vi "Public Key File Authentication.vi"() -> ()   [LabVIEW 2018]
doc: "Logs into a remote SSH server using a username, Public-Private Key pair, and passphrase if the Public Key was created with one. This is arguably a more secure form of authentication than Password Authenication, but it requires configuration on the remote SSH server and/or CompactRIO."
uses:
  Toolkit/Session/Type Definitions/Host Key Hash Types.ctl
  Toolkit/Session/Support/Create from SSH.vi
  Toolkit/Session/Support/Destroy to SSH.vi
  Toolkit/SSH/SSH.lvclass
  Toolkit/Session/Session.lvclass
panel:
  in  "Private Key File":path
  in  "Public Key File":path
  out "Remote Host Key Type":string
  out "Remote Host Key":string
  out "Remote Fingerprint Hash":string
  out "Authenticated":bool
  in  "Remote SSH Server":string
  in  "Passphrase":string
  in  "Username":string
  # "Overview: Demonstrates transferring, or uploading, a local file to a remote SSH server, similar to the SCP command line utility\nInstructions:\n1. Enter the IP address or host name of the remote SSH server. This can be a CompactRIO (cRIO) running the National Instruments Linux Real-Time (NI Linux RT) operating system with the Enable Secure Shell Server (sshd) checkbox checked. \n2. Select a Public Key on the local computer.\n3. Select the Private Key sibling to the Public Key. Note, the Private Key should be private and only accessible by the current, local user. It is best practice to have permissions for the Private Key file be only read/write accessible by the local user and no one else. It is even better to use a key store application for storage of Public-Private Key pairs.\n4. Enter a username. If using a cRIO with a default configuration, then the username is \"admin\".\n5. Enter a passphrase if the Public Key was created with one. Note, it is best practice to always create a public key with a passphrase, then use a SSH agent or key store to only have to use the passphrase on first use of the Public Key for authentication.\n6. Run this VI."
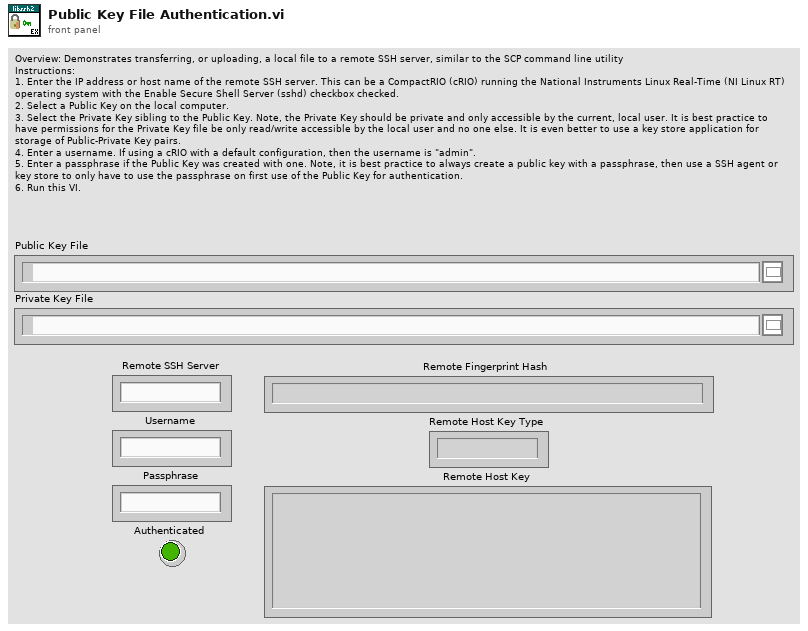
[diagram p1: front panel]
types:
  T1 = typedef "Toolkit.lvlib/Session.lvclass/Host Key Hash Types.ctl" = i32
  T2 = typedef "Toolkit.lvlib/Session.lvclass/Host Key Types.ctl" = i32
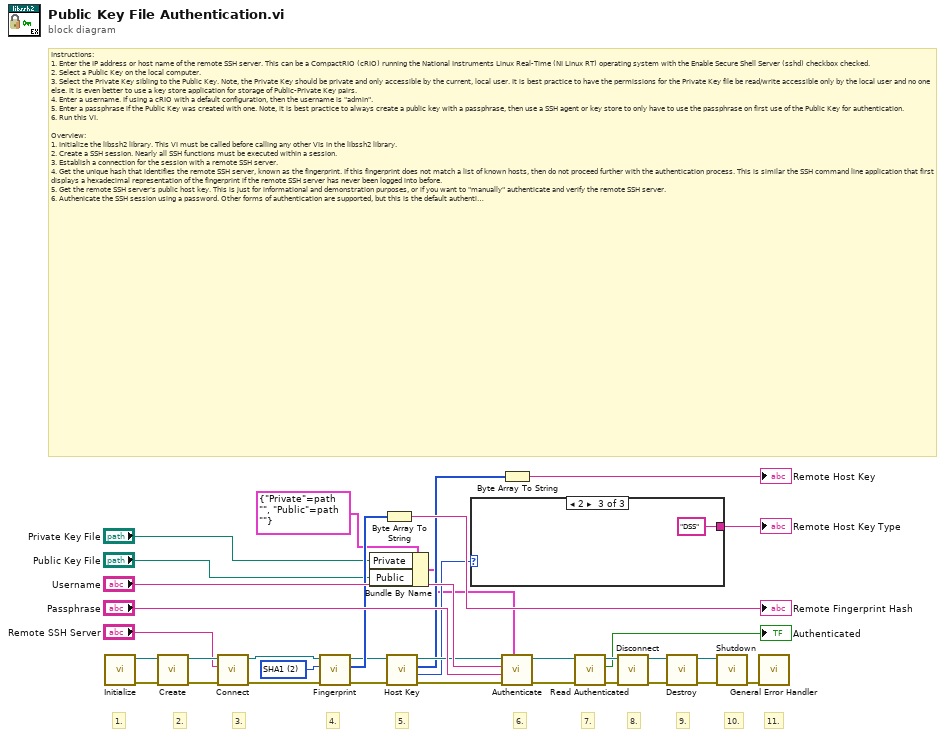
[diagram p0: block diagram]
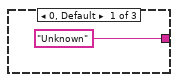
[diagram p2: hidden frame]
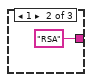
[diagram p3: hidden frame]
diagram:
  w15 = T1 2 items=["MD5"=1, "SHA1"=2] ("Type")
  # "11."
  # "10."
  # "9."
  # "8."
  # "7."
  # "6."
  # "5."
  # "4."
  # "3."
  # "2."
  # "1."
  # "Instructions:\n1. Enter the IP address or host name of the remote SSH server. This can be a CompactRIO (cRIO) running the National Instruments Linux Real-Time (NI Linux RT) operating system with the Enable Secure Shell Server (sshd) checkbox checked. \n2. Select a Public Key on the local computer.\n3. Select the Private Key sibling to the Public Key. Note, the Private Key should be private and only accessible by the current, local user. It is best practice to have the permissions for the Private Key file be read/write accessible only by the local user and no one else. It is even better to use a key store application for storage of Public-Private Key pairs.\n4. Enter a username. If using a cRIO with a default configuration, then the username is \"admin\".\n5. Enter a passphrase if the Public Key was created with one. Note, it is best practice to always create a public key with a passphrase, then use a SSH agent or key store to only have to use the passphrase on first use of the Public Key for authentication.\n6. Run this VI.\n\nOverview:\n1. Initialize the libssh2 library. This VI must be called before calling any other VIs in the libssh2 library.\n2. Create a SSH session. Nearly all SSH functions must be executed within a session.\n3. Establish a connection for the session with a remote SSH server.\n4. Get the unique hash that identifies the remote SSH server, known as the fingerprint. If this fingerprint does not match a list of known hosts, then do not proceed further with the authentication process. This is similar the SSH command line application that first displays a hexadecimal representation of the fingerprint if the remote SSH server has never been logged into before.\n5. Get the remote SSH server's public host key. This is just for informational and demonstration purposes, or if you want to \"manually\" authenticate and verify the remote SSH server.\n6. Authenicate the SSH session using a password. Other forms of authentication are supported, but this is the default authentication scheme for a cRIO. \n7. Check to see if the username and password combination worked to log into the remote SSH server\n8. Disconnect from the remote SSH server.\n9. Destroy the session to free resources within the libssh2 library.\n10. Shutdown the libssh2 library. This VI must be last VI called for the libssh2 library. No other libssh2 VIs should be called once this VI is executed.\n11. Provide some error handling and reporting. Libssh2 errors will be in the -8100 range."
  n1 = call "Initialize.vi"() -> ("Error Out"=w33:errorcluster, "SSH"=w34:refnum<class "SSH.lvclass">)  [unwired: 10 in]
  n2 = call-poly "Create.vi"("Error In"=w33, "SSH"=w34) -> ("Error Out"=w31:errorcluster, "Sesssion"=w32:refnum<class "Session.lvclass">)  [unwired: 8 in]
  n3 = call "Connect.vi"("Error In"=w31, "Address"="Remote SSH Server", "Session In"=w32) -> ("Error Out"=w16:errorcluster, "Sesssion Out"=w17:refnum<class "Session.lvclass">)  [unwired: 7 in]
  n4 = call "Fingerprint.vi"("Error In"=w16, "Type"=w15, "Session In"=w17) -> ("Error Out"=w11:errorcluster, "Fingerprint"=w14:u8[], "Sesssion Out"=w12:refnum<class "Session.lvclass">)  [unwired: 6 in]
  n5 = Bundle By Name(cluster=cluster{"Private":path, "Public":path} {"Private"=path "", "Public"=path ""} ("Keys"), "Private"="Private Key File", "Public"="Public Key File") -> (w1:cluster{"Private":path, "Public":path})
  n6 = Byte Array To String(unsigned byte array=w14) -> (string=→"Remote Fingerprint Hash":string)
  n7 = call "Host Key.vi"("Error In"=w11, "Session In"=w12) -> ("Error Out"=w10:errorcluster, "Type"=w6:T2, "Host Key"=w8:u8[], "Sesssion Out"=w9:refnum<class "Session.lvclass">)  [unwired: 6 in]
  n8 = case shown="2" w6 {
    tunnel: ["Unknown" "RSA" "DSS"] -> w5
    frame 0, Default {
    }
    frame 1 {
    }
    frame 2 {
    }
  }
  "Remote Host Key Type" <- w5
  n9 = Byte Array To String(unsigned byte array=w8) -> (string=→"Remote Host Key":string)
  n10 = call-poly "Authenticate.vi"("Keys"=w1, "Error In"=w10, "Passphrase"="Passphrase", "Username"="Username", "Session In"=w9) -> ("Error Out"=w22:errorcluster, "Sesssion Out"=w21:refnum<class "Session.lvclass">)  [unwired: 5 in]
  n11 = call "Read Authenticated.vi"("Error In"=w22, "Session In"=w21) -> ("Error Out"=w20:errorcluster, "Authenticated"=→"Authenticated":bool, "Sesssion Out"=w19:refnum<class "Session.lvclass">)  [unwired: 7 in]
  n12 = call "Disconnect.vi"("Error In"=w20, "Session In"=w19) -> ("Error Out"=w26:errorcluster, "Sesssion Out"=w27:refnum<class "Session.lvclass">)  [unwired: 8 in]
  n13 = call-poly "Destroy.vi"("Error In"=w26, "Session"=w27) -> ("Error Out"=w24:errorcluster, "SSH"=w25:refnum<class "SSH.lvclass">)  [unwired: 8 in]
  n14 = call "Shutdown.vi"("Error In"=w24, "SSH"=w25) -> ("Error Out"=w23:errorcluster)  [unwired: 9 in]
  n15 = call <vilib>:"General Error Handler.vi"("error in (no error)"=w23) -> ()  [unwired: 10 in, 5 out]
